vi "Test_DO-port.vi"() -> ()   [LabVIEW 2019]
uses:
  <vilib>/DAQmx/write.llb/DAQmx Write (Digital 1D Bool NChan 1Samp 1Line).vi
  <vilib>/DAQmx/create/channels.llb/DAQmx Create Channel (DO-Digital Output).vi
  <vilib>/DAQmx/miscellaneous.llb/DAQmx Fill In Error Info.vi
panel:
  out "error out":errorcluster
  in  "data":bool[](array[boolean])=[FALSE, FALSE, FALSE, FALSE, FALSE, FALSE, FALSE, FALSE, FALSE, FALSE, FALSE, FALSE, FALSE, FALSE, FALSE, FALSE, FALSE, FALSE, FALSE, FALSE, FALSE, FALSE, FALSE, FALSE, FALSE, FALSE, FALSE, FALSE, FALSE, FALSE, FALSE, FALSE]
  in  "lines":tag="cDAQ9185-213AA55Mod1/port0"
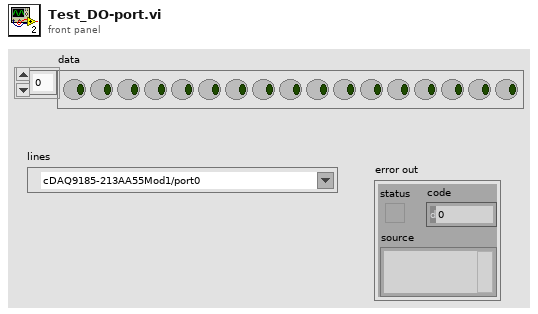
[diagram p1: front panel]
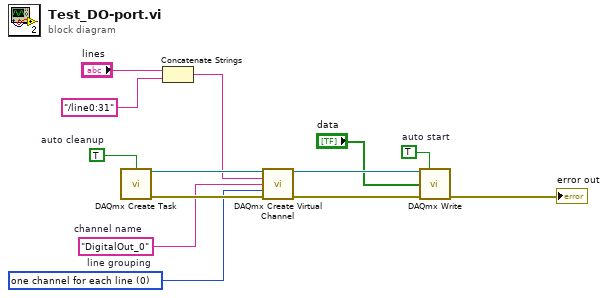
[diagram p0: block diagram]
diagram:
  w9 = TRUE  # auto cleanup
  w7 = 0 items=["one channel for each line", "one channel for all lines"]  # line grouping
  w8 = "DigitalOut_0"  # channel name
  w6 = TRUE  # auto start
  n1 = call <vilib>:"DAQmx Create Task.vi"("auto cleanup"=w9) -> ("task out"=w11:refnum<k21>, "error out"=w10:errorcluster)  [unwired: 13 in]
  n2 = Concatenate Strings("lines", "/line0:31" ("string")) -> (w1:string)
  n3 = call-poly <vilib>:"DAQmx Create Virtual Channel.vi"("task in"=w11, "lines"=w1, "name to assign"=w8, "line grouping"=w7, "error in"=w10) -> ("task out"=w12:refnum<k21>, "error out"=w13:errorcluster)  [unwired: 9 in]
  n4 = call-poly <vilib>:"DAQmx Write.vi"("task/channels in"=w12, "auto start"=w6, "data"="data", "error in"=w13) -> ("error out"=→"error out":errorcluster)  [unwired: 9 in, 2 out]
